vi "test Timestamps with Start and Stop Command.vi"(8 "error in":errorcluster, 11 "Loopback in":refnum<class "Loopback.lvclass">) -> (0 "error out":errorcluster, 3 "Loopback out":refnum<class "Loopback.lvclass">)   [LabVIEW 2020, in "Loopback.lvclass"]
uses:
  Loopback.lvclass
  <vilib>/NI VeriStand/Execution/Workspace/NI_VS Workspace ExecutionAPI.lvlib
  <vilib>/NI VeriStand/Execution/Workspace/NI VeriStand - Set Single Channel Value.vi
  d018f213-e546-4c43-981e-280bd99d7f58.vi
  <vilib>/addons/_JKI Toolkits/VI Tester/TestCase.llb/TestCase.lvclass
  <vilib>/NI/VeriStand Custom Device Testing Tools/VeriStandTestUtilities/VeriStandTestUtilities.lvlib
  862773ac-e8dc-46d6-a348-dc8e2e4002c1.vi
  <vilib>/numeric/Random Number (Range) U64.vi
  Shared/Running Status.ctl
  <vilib>/NI VeriStand/Execution/Workspace/NI VeriStand - Get Single Channel Value.vi
  C:/Program Files (x86)/National Instruments/LabVIEW 2020/vi.lib/addons/_JKI Toolkits/VI Tester/TestCase.llb/TestCase.lvclass
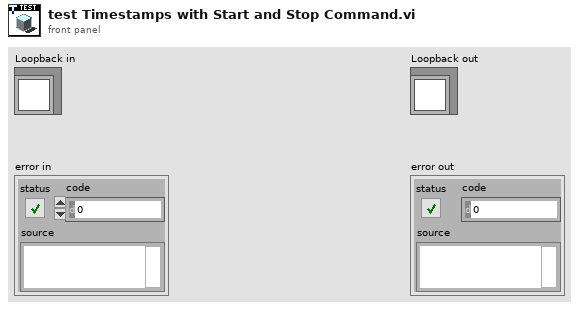
[diagram p1: front panel]
types:
  T1 = typedef "Running Status.ctl" = enum16{"Running", "Stopped"}
  T2 = typedef "NI_VS Workspace ExecutionAPI.lvlib/WorkspaceAPI.ctl" = refnum<k24>
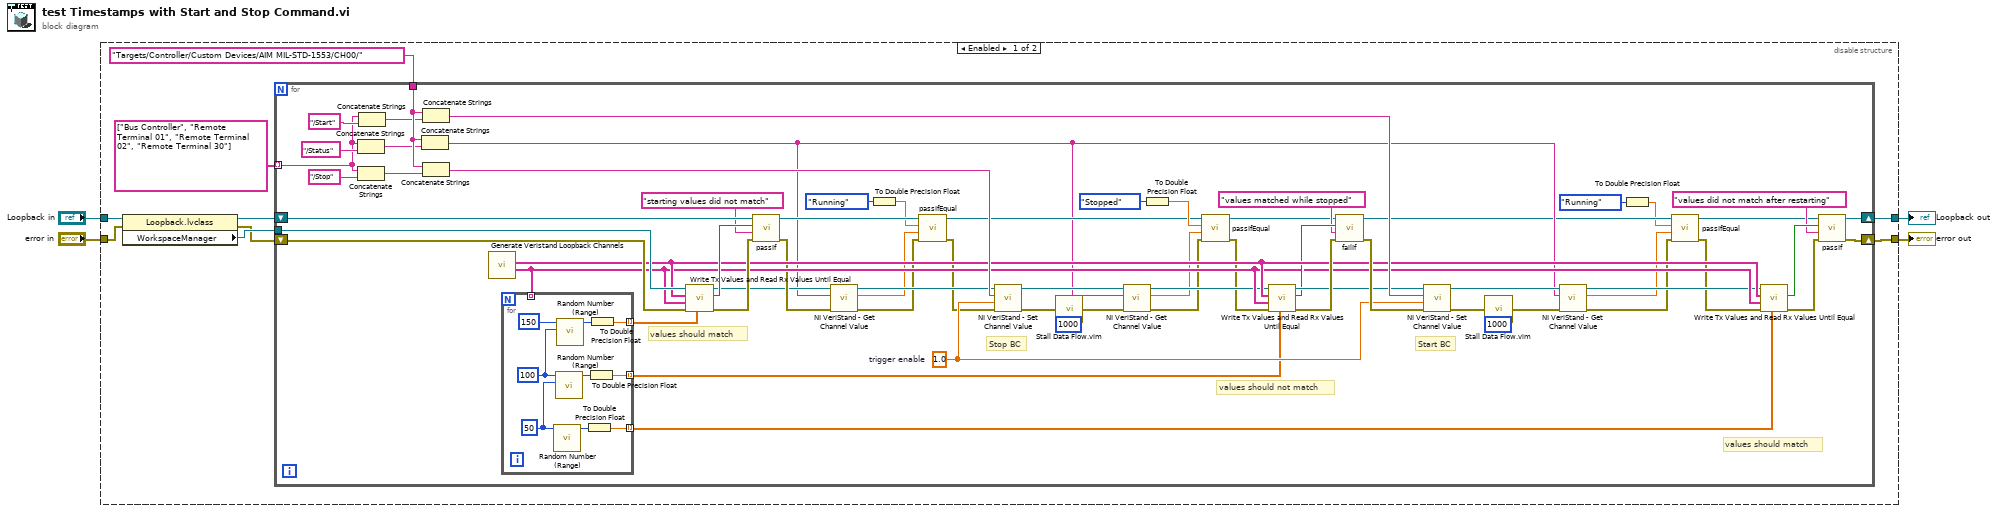
[diagram p0: block diagram]
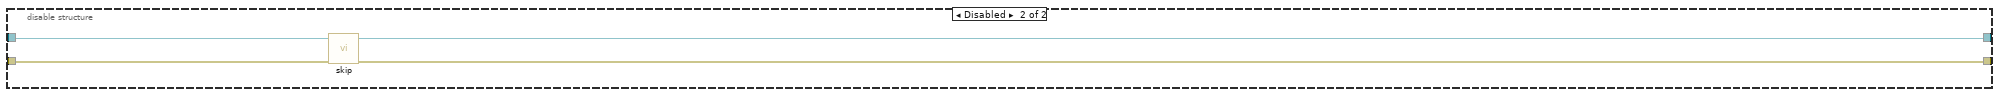
[diagram p2: hidden frame]
diagram:
  n1 = disable-structure shown="Enabled" {
    disable-tunnel: [w12 w90] -> w4
    disable-tunnel: [w13 w89] -> w1
    disable-tunnel: "Loopback in" -> [w11 w91]
    disable-tunnel: "error in" -> [w10 w92]
    frame Enabled {
      n2 = property class="Loopback.lvclass"(reference=w11, error in=w10) -> (reference out=w9:refnum<class "Loopback.lvclass">, error out=w7:errorcluster, "WorkspaceManager"=w8:T2)
      n3 = for {
        tunnel: w8 -> [w71]
        tunnel: "Targets/Controller/Custom Devices/AIM MIL-STD-1553/CH00/" ("base name for channel aliases") -> [w50]
        shift-right: [w77] -> w13
        shift-left: w9 -> [w72]
        shift-right: [w76] -> w12
        shift-left: w7 -> [w70]
        tunnel: string[] ["Bus Controller", "Remote Terminal 01", "Remote Terminal 02", "Remote Terminal 30"] -> [w14] mode=indexing
        w63 = 1.0  # trigger enable
        # "values should match"
        # "Start BC"
        # "values should not match"
        # "Stop BC"
        # "values should match"
        n4 = Concatenate Strings(w14, "/Status" ("Channel")) -> (w16:string)
        n5 = Concatenate Strings(w14, "/Stop" ("Channel")) -> (w17:string)
        n6 = Concatenate Strings(w14, "/Start" ("Channel")) -> (w15:string)
        n7 = Concatenate Strings(w50, w16) -> (w29:string)
        n8 = Concatenate Strings(w50, w15) -> (w78:string)
        n9 = Concatenate Strings(w50, w17) -> (w79:string)
        n10 = call "Generate Veristand Loopback Channels.vi"() -> ("Rx Aliases"=w55:string[], "Tx Aliases"=w61:string[])  [unwired: 10 in]
        n11 = for {
          tunnel: [w86] -> w60 mode=indexing
          tunnel: [w81] -> w58 mode=indexing
          tunnel: [w80] -> w59 mode=indexing
          tunnel: w55 -> [_] mode=indexing
          w83 = u64 50 ("upper bound (100)")
          w82 = u64 100 ("upper bound (100)")
          n12 = call-poly <vilib>:"Random Number (Range).vi"("upper bound (100)"=w83) -> ("number"=w84:u64)  [unwired: 10 in]
          n13 = call-poly <vilib>:"Random Number (Range).vi"("lower bound (0)"=w83, "upper bound (100)"=w82) -> ("number"=w85:u64)  [unwired: 9 in]
          n14 = call-poly <vilib>:"Random Number (Range).vi"("lower bound (0)"=w82, "upper bound (100)"=u64 150) -> ("number"=w88:u64)  [unwired: 9 in]
          n15 = To Double Precision Float(number=w84) -> (double precision float=w81:dbl)
          n16 = To Double Precision Float(number=w85) -> (double precision float=w80:dbl)
          n17 = To Double Precision Float(number=w88) -> (double precision float=w86:dbl)
        }
        n18 = call <vilib>:"Write Tx Values and Read Rx Values Until Equal.vi"("Tx values"=w60, "error in"=w70, "Rx aliases"=w55, "Tx aliases"=w61, "workspace manager in"=w71) -> ("error out"=w69:errorcluster, "values equal"=w62:bool, "workspace manager out"=w45:T2)  [unwired: 4 in]
        n19 = call-dynamic "passIf.vi"("error in (no error)"=w69, "message (\"\")"="starting values did not match" ("message (\"\")"), "pass"=w62, "TestCase in"=w72) -> ("error out"=w47:errorcluster, "TestCase out"=w43:refnum<class "Loopback.lvclass">)  [unwired: 6 in]
        n20 = call-poly <vilib>:"NI VeriStand - Get Channel Value.vi"("error in (no error)"=w47, "Channel"=w29, "WorkspaceManager in"=w45) -> ("error out"=w40:errorcluster, "Value"=w41:dbl, "WorkspaceManager out"=w46:T2)  [unwired: 6 in]
        n21 = To Double Precision Float(number=Running_Status."Running" ("Running Status")) -> (double precision float=w42:dbl)
        n22 = call-dynamic "passIfEqual.vi"("error in (no error)"=w40, "y"=w41, "x"=w42, "TestCase in"=w43) -> ("error out"=w39:errorcluster, "TestCase out"=w34:refnum<class "Loopback.lvclass">)  [unwired: 6 in]
        n23 = call-poly <vilib>:"NI VeriStand - Set Channel Value.vi"("error in (no error)"=w39, "Value"=w63, "Channel"=w79, "WorkspaceManager in"=w46) -> ("error out"=w73:errorcluster, "WorkspaceManager out"=w49:T2)  [unwired: 6 in]
        n24 = call "Stall Data Flow.vim"("value in"=w73, "milliseconds to wait"=u32 1000) -> ("value out"=w51:errorcluster)  [unwired: 1 out]
        n25 = call-poly <vilib>:"NI VeriStand - Get Channel Value.vi"("error in (no error)"=w51, "Channel"=w29, "WorkspaceManager in"=w49) -> ("error out"=w38:errorcluster, "Value"=w37:dbl, "WorkspaceManager out"=w48:T2)  [unwired: 6 in]
        n26 = To Double Precision Float(number=Running_Status."Stopped" ("Running Status")) -> (double precision float=w35:dbl)
        n27 = call-dynamic "passIfEqual.vi"("error in (no error)"=w38, "y"=w37, "x"=w35, "TestCase in"=w34) -> ("error out"=w33:errorcluster, "TestCase out"=w32:refnum<class "Loopback.lvclass">)  [unwired: 6 in]
        n28 = call <vilib>:"Write Tx Values and Read Rx Values Until Equal.vi"("Tx values"=w59, "error in"=w33, "Rx aliases"=w55, "Tx aliases"=w61, "workspace manager in"=w48) -> ("error out"=w68:errorcluster, "values equal"=w56:bool, "workspace manager out"=w67:T2)  [unwired: 4 in]
        n29 = call-dynamic "failIf.vi"("error in (no error)"=w68, "message (\"\")"="values matched while stopped" ("message (\"\")"), "fail"=w56, "TestCase in"=w32) -> ("error out"=w75:errorcluster, "TestCase out"=w24:refnum<class "Loopback.lvclass">)  [unwired: 6 in]
        n30 = call-poly <vilib>:"NI VeriStand - Set Channel Value.vi"("error in (no error)"=w75, "Value"=w63, "Channel"=w78, "WorkspaceManager in"=w67) -> ("error out"=w65:errorcluster, "WorkspaceManager out"=w30:T2)  [unwired: 6 in]
        n31 = call "Stall Data Flow.vim"("value in"=w65, "milliseconds to wait"=u32 1000) -> ("value out"=w31:errorcluster)  [unwired: 1 out]
        n32 = call-poly <vilib>:"NI VeriStand - Get Channel Value.vi"("error in (no error)"=w31, "Channel"=w29, "WorkspaceManager in"=w30) -> ("error out"=w27:errorcluster, "Value"=w21:dbl, "WorkspaceManager out"=w28:T2)  [unwired: 6 in]
        n33 = To Double Precision Float(number=Running_Status."Running" ("Running Status")) -> (double precision float=w22:dbl)
        n34 = call-dynamic "passIfEqual.vi"("error in (no error)"=w27, "y"=w21, "x"=w22, "TestCase in"=w24) -> ("error out"=w26:errorcluster, "TestCase out"=w25:refnum<class "Loopback.lvclass">)  [unwired: 6 in]
        n35 = call <vilib>:"Write Tx Values and Read Rx Values Until Equal.vi"("Tx values"=w58, "error in"=w26, "Rx aliases"=w55, "Tx aliases"=w61, "workspace manager in"=w28) -> ("error out"=w64:errorcluster, "values equal"=w57:bool)  [unwired: 4 in, 1 out]
        n36 = call-dynamic "passIf.vi"("error in (no error)"=w64, "message (\"\")"="values did not match after restarting" ("message (\"\")"), "pass"=w57, "TestCase in"=w25) -> ("error out"=w76:errorcluster, "TestCase out"=w77:refnum<class "Loopback.lvclass">)  [unwired: 6 in]
      }
    }
    frame Disabled {
      n37 = call <vilib>:"skip.vi"("error in (no error)"=w92, "TestCase in"=w91) -> ("error out"=w90:errorcluster, "TestCase out"=w89:refnum<class "Loopback.lvclass">)  [unwired: 8 in]
    }
  }
  "error out" <- w4
  "Loopback out" <- w1
